vi "Laser-Power-Loop.vi"(7 "Steps":u8, 8 "AOTF-Analog Max Voltage":dbl, 9 "AOTF-Analog Min Voltage":dbl, 10 "Last Intensity":i8, 11 "First Intensity":i8) -> (2 "Power":dbl[](array[numeric]), 3 "Power-Absolute":dbl[](array[numeric]))   [LabVIEW 2009]
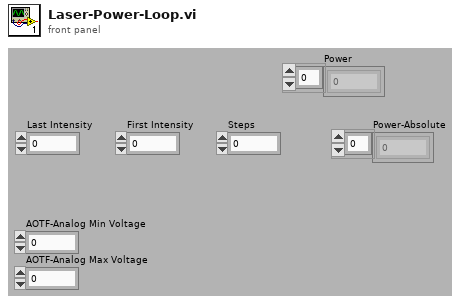
[diagram p1: front panel]
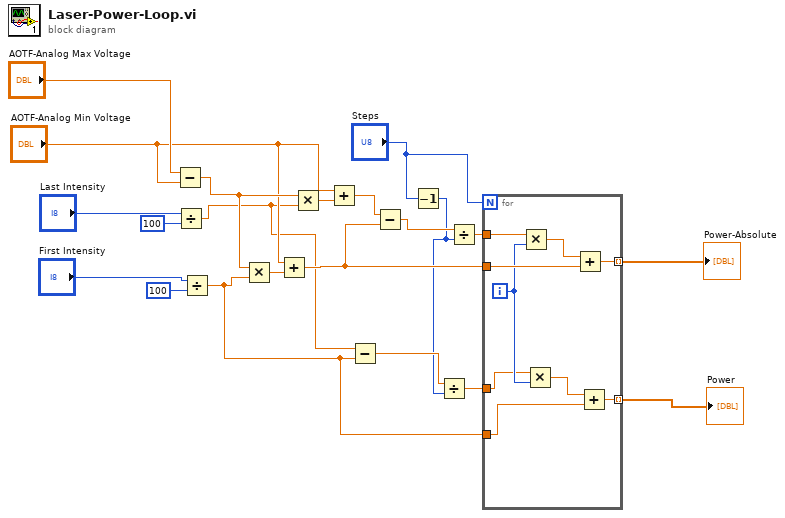
[diagram p0: block diagram]
diagram:
  n1 = Subtract(x="AOTF-Analog Max Voltage", y="AOTF-Analog Min Voltage") -> (x-y=w17:dbl)
  n2 = Divide(x="Last Intensity", y=i8 100) -> (x/y=w8:dbl)
  n3 = Divide(x="First Intensity", y=i8 100) -> (x/y=w2:dbl)
  n4 = Multiply(x=w17, y=w2) -> (x*y=w7:dbl)
  n5 = Add(x="AOTF-Analog Min Voltage", y=w7) -> (x+y=w14:dbl)
  n6 = Multiply(x=w17, y=w8) -> (x*y=w20:dbl)
  n7 = Add(x="AOTF-Analog Min Voltage", y=w20) -> (x+y=w16:dbl)
  n8 = Subtract(x=w8, y=w2) -> (x-y=w6:dbl)
  n9 = Subtract(x=w16, y=w14) -> (x-y=w15:dbl)
  n10 = Decrement(x="Steps") -> (x-1=w5:u8)
  n11 = Divide(x=w6, y=w5) -> (x/y=w4:dbl)
  n12 = Divide(x=w15, y=w5) -> (x/y=w13:dbl)
  n13 = for {
    N: "Steps" -> [_]
    tunnel: [w27] -> w9 mode=indexing
    tunnel: w14 -> [w28]
    tunnel: w13 -> [w30]
    tunnel: w2 -> [w23]
    tunnel: w4 -> [w24]
    tunnel: [w22] -> w1 mode=indexing
    i -> [w25]
    n14 = Multiply(x=w30, y=w25) -> (x*y=w29:dbl)
    n15 = Multiply(x=w24, y=w25) -> (x*y=w26:dbl)
    n16 = Add(x=w29, y=w28) -> (x+y=w27:dbl)
    n17 = Add(x=w26, y=w23) -> (x+y=w22:dbl)
  }
  "Power-Absolute" <- w9
  "Power" <- w1
